vi "Ping Pong Data between BRAM.vi"(5 "Read Count":u16, 7 "Write Count":u16, 8 "Input Valid":bool, 10 "Bank1 Data":T1, 11 "Bank0 Data":T2) -> (0 "Read Valid":bool, 2 "Address1. Element Out":u16, 3 "Address0. Element Out":u16)   [LabVIEW 2012]
doc: "This VI does ping pong between two BRAM blocks\n\n<b> Latency = 3 Ticks </b>"
uses:
  <vilib>/rvi/FXPMathLib/basic elements/FxpDiscreteDelay/XNode/nifxpmath_DiscreteDelay.xnode
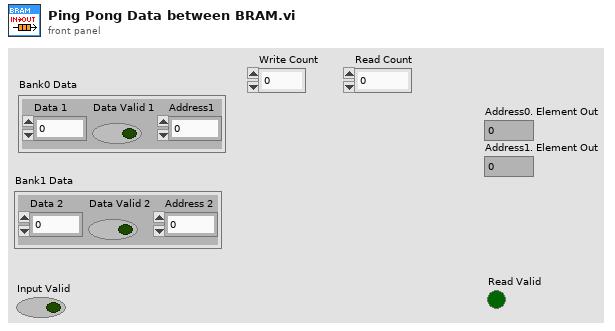
[diagram p1: front panel]
types:
  T1 = cluster{"Data 2":u16, "Data Valid 2":bool, "Address 2":u16}
  T2 = cluster{"Data 1":u16, "Data Valid 1":bool, "Address1":u16}
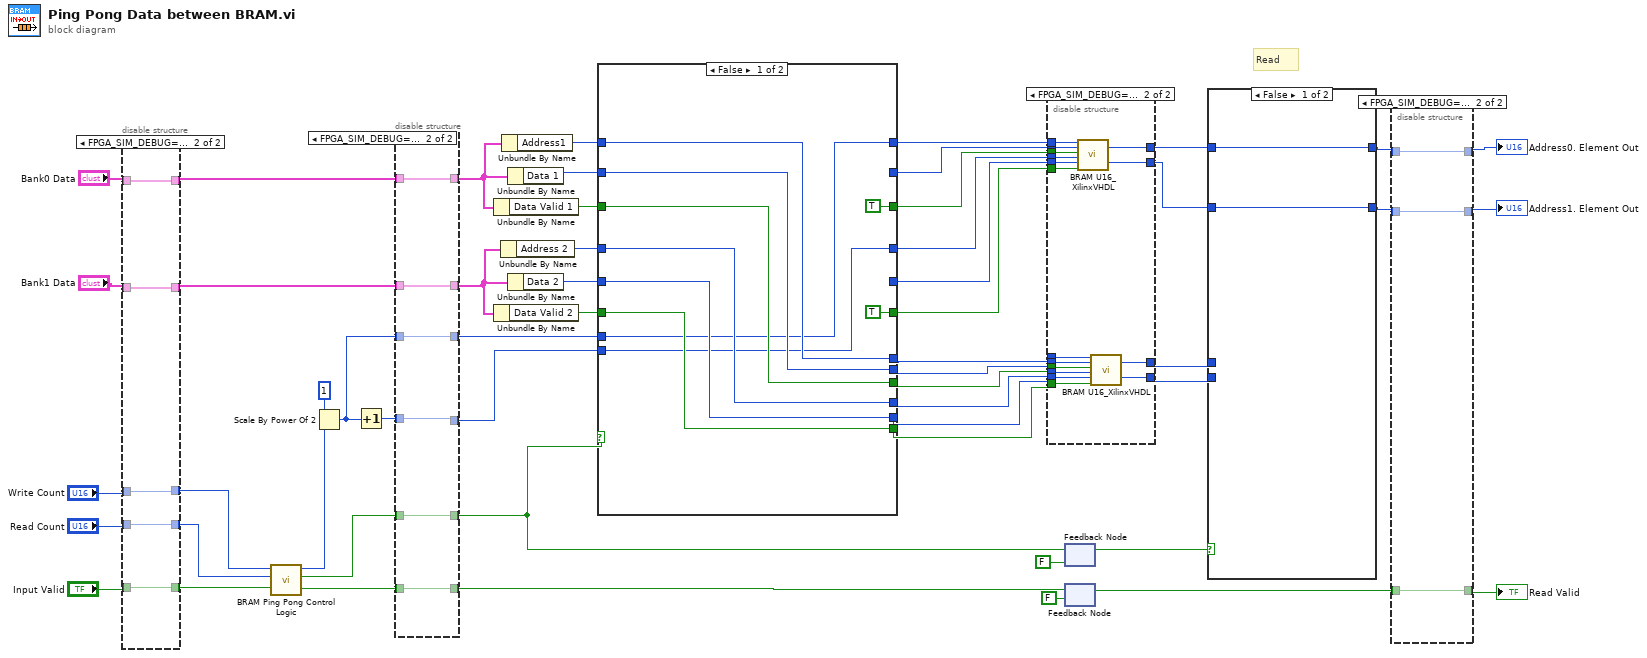
[diagram p0: block diagram]
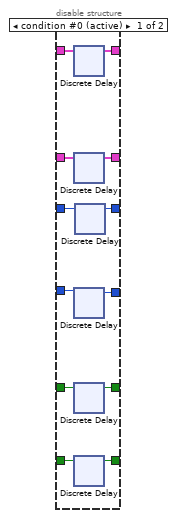
[diagram p2: hidden frame]
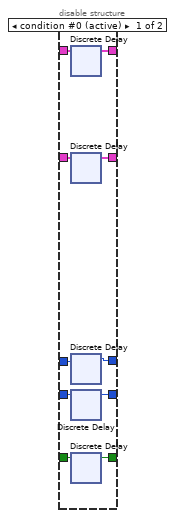
[diagram p3: hidden frame]
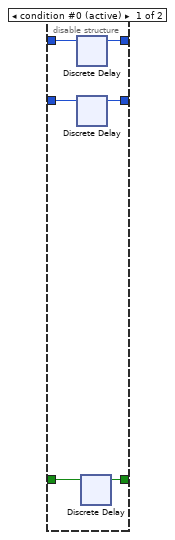
[diagram p4: hidden frame]
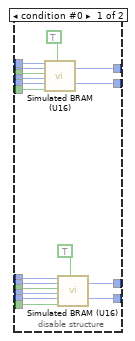
[diagram p5: hidden frame]
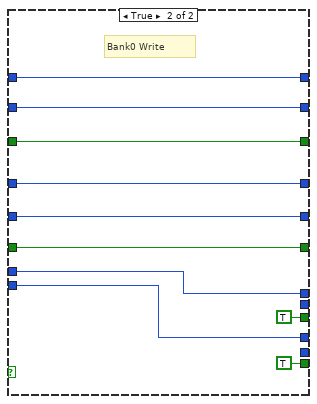
[diagram p7: hidden frame]
diagram:
  # "Read"
  n1 = disable-structure shown="FPGA_SIM_DEBUG==TRUE" {
    disable-tunnel: "Bank0 Data" -> [w63 w68]
    disable-tunnel: "Bank1 Data" -> [w62 w67]
    disable-tunnel: "Input Valid" -> [w61 w64]
    disable-tunnel: "Write Count" -> [w60 w66]
    disable-tunnel: "Read Count" -> [w59 w65]
    disable-tunnel: [w58 w68] -> w15
    disable-tunnel: [w57 w67] -> w14
    disable-tunnel: [w56 w64] -> w13
    disable-tunnel: [w55 w66] -> w9
    disable-tunnel: [w54 w65] -> w8
    frame condition #0 (active) {
      n2 = xnode "Discrete Delay"("D"=w63) -> ("Q"=w58:T2)
      n3 = xnode "Discrete Delay"("D"=w62) -> ("Q"=w57:T1)
      n4 = xnode "Discrete Delay"("D"=w60) -> ("Q"=w55:u16)
      n5 = xnode "Discrete Delay"("D"=w59) -> ("Q"=w54:u16)
      n6 = xnode "Discrete Delay"("D"=w61) -> ("Q"=w56:bool)
    }
    frame condition #1 {
    }
  }
  n7 = call <userlib>:"BRAM Ping Pong Control Logic.vi"("Input Valid"=w13, "Read Count"=w8, "Write Count"=w9) -> ("Read Valid"=w26:bool, "BRAM Bank0 Write?"=w20:bool, "Read Address"=w21:u16)  [unwired: 6 in]
  n8 = Scale By Power Of 2(n=1, x=w21) -> (x*2^n=w2:u16)
  n9 = Increment(x=w2) -> (x+1=w24:u16)
  n10 = disable-structure shown="FPGA_SIM_DEBUG==TRUE" {
    disable-tunnel: w26 -> [w80 w81]
    disable-tunnel: w24 -> [w79 w83]
    disable-tunnel: w20 -> [w78 w82]
    disable-tunnel: w15 -> [w77 w86]
    disable-tunnel: w14 -> [w76 w85]
    disable-tunnel: [w75 w83] -> w7
    disable-tunnel: [w74 w85] -> w6
    disable-tunnel: [w73 w86] -> w5
    disable-tunnel: [w72 w82] -> w4
    disable-tunnel: [w71 w81] -> w3
    disable-tunnel: w2 -> [w70 w84]
    disable-tunnel: [w69 w84] -> w1
    frame condition #0 (active) {
      n11 = xnode "Discrete Delay"("D"=w77) -> ("Q"=w73:T2)
      n12 = xnode "Discrete Delay"("D"=w76) -> ("Q"=w74:T1)
      n13 = xnode "Discrete Delay"("D"=w79) -> ("Q"=w75:u16)
      n14 = xnode "Discrete Delay"("D"=w78) -> ("Q"=w72:bool)
      n15 = xnode "Discrete Delay"("D"=w80) -> ("Q"=w71:bool)
      n16 = xnode "Discrete Delay"("D"=w70) -> ("Q"=w69:u16)
    }
    frame condition #1 {
    }
  }
  n17 = Unbundle By Name(w5) -> ("Data Valid 1"=w42:bool)
  n18 = Unbundle By Name(w6) -> ("Data Valid 2"=w35:bool)
  n19 = Unbundle By Name(w6) -> ("Address 2"=w39:u16)
  n20 = Unbundle By Name(w5) -> ("Address1"=w45:u16)
  n21 = Unbundle By Name(w5) -> ("Data 1"=w46:u16)
  n22 = Unbundle By Name(w6) -> ("Data 2"=w38:u16)
  n23 = case shown="False" w4 {
    tunnel: w46 -> [w95 w105]
    tunnel: w42 -> [w94 w104]
    tunnel: [_ w105] -> w53
    tunnel: w45 -> [w96 w106]
    tunnel: [w88 w106] -> w44
    tunnel: [TRUE ("Data Valid 1") w104] -> w40
    tunnel: w39 -> [w93 w103]
    tunnel: [w87 w103] -> w37
    tunnel: w38 -> [w92 w102]
    tunnel: [_ w102] -> w36
    tunnel: w35 -> [w91 w101]
    tunnel: [TRUE ("Data Valid 2") w101] -> w34
    tunnel: [w96 w98] -> w33
    tunnel: [w95 _] -> w32
    tunnel: [w94 TRUE ("Data Valid 1")] -> w31
    tunnel: [w93 w97] -> w30
    tunnel: [w92 _] -> w29
    tunnel: [w91 TRUE ("Data Valid 2")] -> w28
    tunnel: w1 -> [w88 w98]
    tunnel: w7 -> [w87 w97]
    frame False {
    }
    frame True {
      # "Bank0 Write"
    }
  }
  n24 = disable-structure shown="FPGA_SIM_DEBUG==FALSE, default" {
    disable-tunnel: w53 -> [w124 w140]
    disable-tunnel: [w123 w139] -> w52
    disable-tunnel: [w122 w138] -> w51
    disable-tunnel: [w121 w137] -> w50
    disable-tunnel: [w120 w136] -> w49
    disable-tunnel: w44 -> [w119 w135]
    disable-tunnel: w40 -> [w118 w134]
    disable-tunnel: w37 -> [w117 w133]
    disable-tunnel: w36 -> [w116 w132]
    disable-tunnel: w34 -> [w115 w131]
    disable-tunnel: w33 -> [w114 w130]
    disable-tunnel: w32 -> [w113 w129]
    disable-tunnel: w31 -> [w112 w128]
    disable-tunnel: w30 -> [w111 w127]
    disable-tunnel: w29 -> [w110 w126]
    disable-tunnel: w28 -> [w109 w125]
    frame condition #0 {
      n25 = call <userlib>:"Simulated BRAM (U16).vi"("Address 0"=w119, "Address0.Element In"=w124, "Address 0 Write"=w118, "Address 1"=w117, "Address1.Element In"=w116, "Address 1 Write"=w115, "Read Before Write?"=TRUE) -> ("Address0. Element Out"=w123:u16, "Address1. Element Out"=w122:u16)  [unwired: 10 in, 1 out]
      n26 = call <userlib>:"Simulated BRAM (U16).vi"("Address 0"=w114, "Address0.Element In"=w113, "Address 0 Write"=w112, "Address 1"=w111, "Address1.Element In"=w110, "Address 1 Write"=w109, "Read Before Write?"=TRUE) -> ("Address0. Element Out"=w121:u16, "Address1. Element Out"=w120:u16)  [unwired: 10 in, 1 out]
    }
    frame condition #1 (active) {
      n27 = call <userlib>:"BRAM U16_XilinxVHDL.vi"("Address 0"=w135, "Address0.Data"=w140, "Address0 Write?"=w134, "Address 1"=w133, "Address1.Data"=w132, "Address1 Write ?"=w131) -> ("Address 0.Element Out"=w139:u16, "Address 1.Element Out"=w138:u16)  [unwired: 12 in]
      n28 = call <userlib>:"BRAM U16_XilinxVHDL.vi"("Address 0"=w130, "Address0.Data"=w129, "Address0 Write?"=w128, "Address 1"=w127, "Address1.Data"=w126, "Address1 Write ?"=w125) -> ("Address 0.Element Out"=w137:u16, "Address 1.Element Out"=w136:u16)  [unwired: 12 in]
    }
  }
  n29 = feedback-in #1(w4) -> ()
  n30 = feedback #1(FALSE ("BRAM Bank0 Write?")) -> (w17:bool)
  n31 = feedback-in #2(w3) -> ()
  n32 = feedback #2(FALSE ("Read Valid")) -> (w19:bool)
  n33 = case shown="False" w17 {
    tunnel: w52 -> [w142 _]
    tunnel: w51 -> [w141 _]
    tunnel: w50 -> [_ w144]
    tunnel: w49 -> [_ w143]
    tunnel: [w142 w144] -> w48
    tunnel: [w141 w143] -> w47
    frame False {
    }
    frame True {
    }
  }
  n34 = disable-structure shown="FPGA_SIM_DEBUG==TRUE" {
    disable-tunnel: w48 -> [w150 w153]
    disable-tunnel: w47 -> [w149 w152]
    disable-tunnel: w19 -> [w148 w151]
    disable-tunnel: [w147 w151] -> w12
    disable-tunnel: [w146 w152] -> w11
    disable-tunnel: [w145 w153] -> w10
    frame condition #0 (active) {
      n35 = xnode "Discrete Delay"("D"=w150) -> ("Q"=w145:u16)
      n36 = xnode "Discrete Delay"("D"=w149) -> ("Q"=w146:u16)
      n37 = xnode "Discrete Delay"("D"=w148) -> ("Q"=w147:bool)
    }
    frame condition #1 {
    }
  }
  "Address0. Element Out" <- w10
  "Address1. Element Out" <- w11
  "Read Valid" <- w12
